vi "Modify Current Mode to String.vi"(8 "Current Mode table":string[][](array[string]), 10 "File Path":path=path "C:/Users/User/Desktop/2023_05_19_14_02.csv", 11 "Data\nNumber":i32) -> ()   [LabVIEW 2023]
uses:
  <vilib>/Utility/file.llb/Read Delimited Spreadsheet (string).vi
  <vilib>/Utility/file.llb/Write Delimited Spreadsheet (string).vi
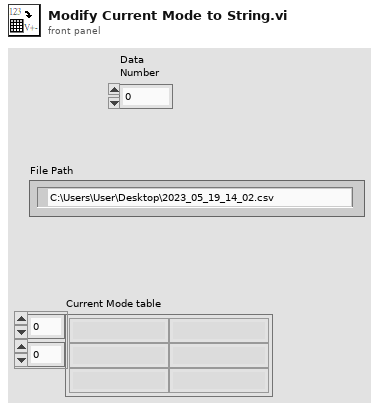
[diagram p1: front panel]
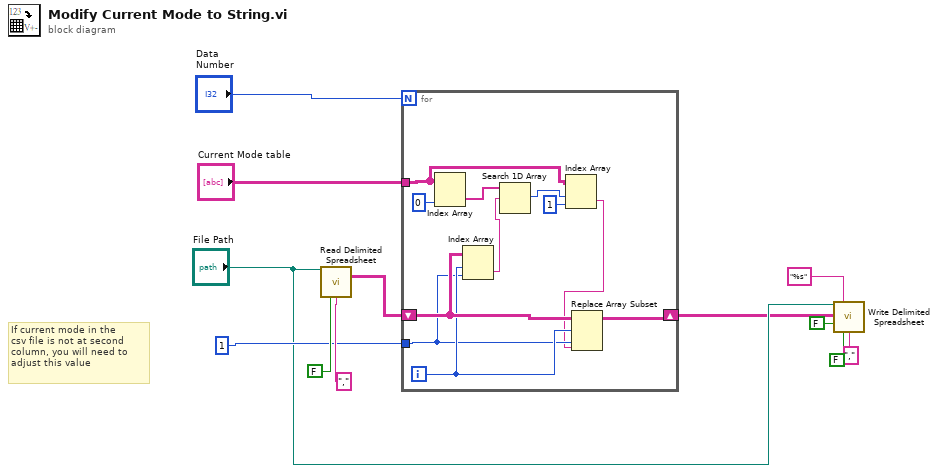
[diagram p0: block diagram]
diagram:
  # "If current mode in the\ncsv file is not at second\ncolumn, you will need to\nadjust this value"
  n1 = call-poly <vilib>:"Read Delimited Spreadsheet.vi"("file path (dialog if empty)"="File Path", "transpose? (F)"=FALSE, "delimiter (\\t)"="," ("delimiter (\\t)")) -> ("all rows"=w10:string[][])  [unwired: 7 in, 5 out]
  n2 = for {
    N: "Data\nNumber" -> [_]
    tunnel: 1 -> [w20]
    shift-right: [w23] -> w1
    shift-left: w10 -> [w22]
    tunnel: "Current Mode table" -> [w15]
    i -> [w21]
    n3 = Index Array(array=w15, index (col)=0 ("disabled index (col)")) -> (element=w18:string[])  [unwired: 1 in]
    n4 = Index Array(array=w22, index (row)=w21, index (col)=w20) -> (element=w17:string)
    n5 = Search 1D Array(1D array=w18, element=w17) -> (index of element=w13:i32)  [unwired: 1 in]
    n6 = Index Array(array=w15, index (row)=w13, index (col)=1) -> (element=w14:string)
    n7 = Replace Array Subset(array=w22, new element=w14, index (row)=w21, index (col)=w20) -> (w23:string[][])
  }
  n8 = call-poly <vilib>:"Write Delimited Spreadsheet.vi"("file path (dialog if empty)"="File Path", "format (%s)"="%s" ("format (%.3f)"), "2D data"=w1, "append to file? (new file:F)"=FALSE, "transpose? (no:F)"=FALSE, "delimiter (\\t)"="," ("delimiter (\\t)")) -> ()  [unwired: 8 in, 2 out]
